vi "故障告警分析.vi"(8 "告警代码":u16, 9 "故障代码":u16, 10 "运行步序":u16, 11 "参数":string) -> (1 "告警记录":T1, 2 "故障记录":T1, 3 "简易报警状态":cluster{"故障状态":string, "报警状态":string})   [LabVIEW 2016, in "斯坦道总磷总氮V2.lvlib"]
panel:
  # "1、注射泵水样阀口堵塞；\n2、注射泵阀过载或丝杆无动作。"
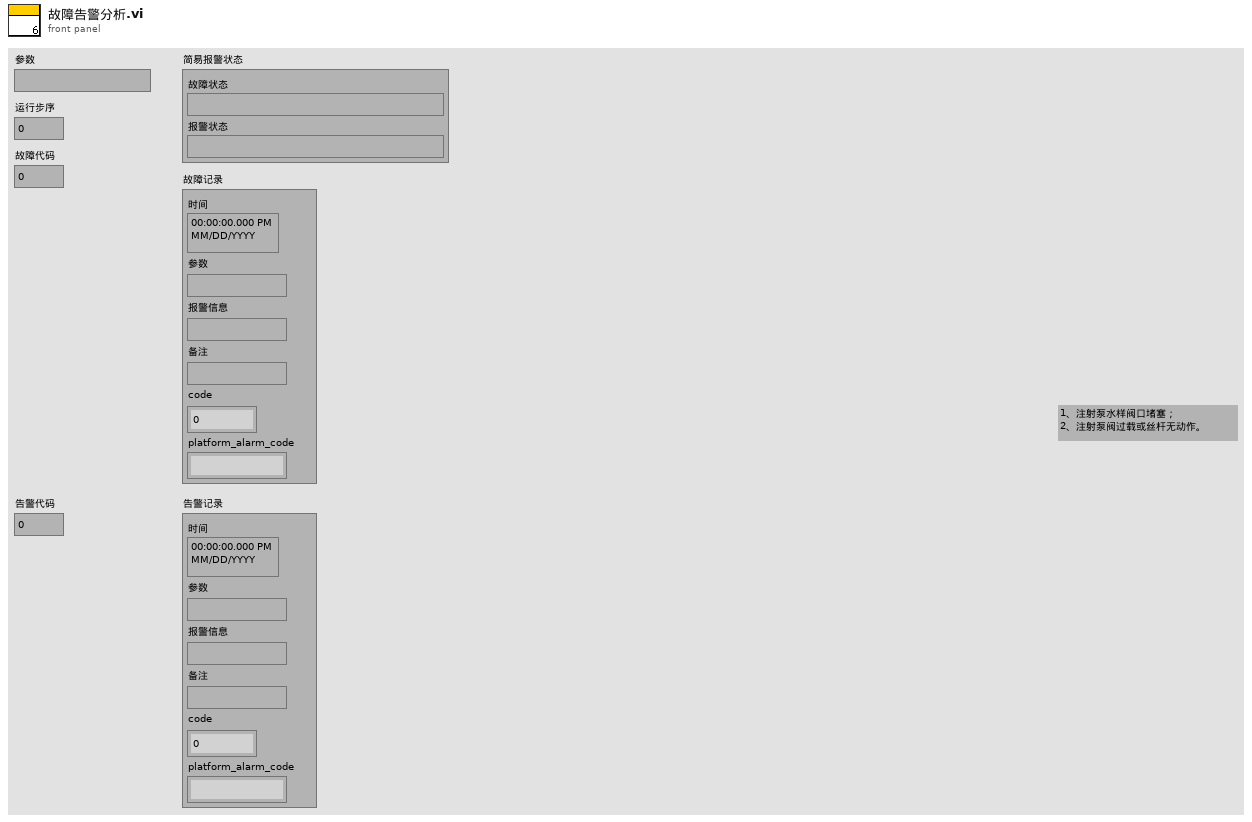
[diagram p1: front panel]
types:
  T1 = typedef "报警信息字段定义.ctl" = cluster{"时间":timestamp, "参数":string, "报警信息":string, "备注":string, "code":u64, "platform_alarm_code":string}
  T2 = cluster{"id":string, "ver":string, "type":string, "code":u16, "level":enum16{"一级", "二级", "三级"}, "message":string, "analysis":string, "platform_alarm_code":string}
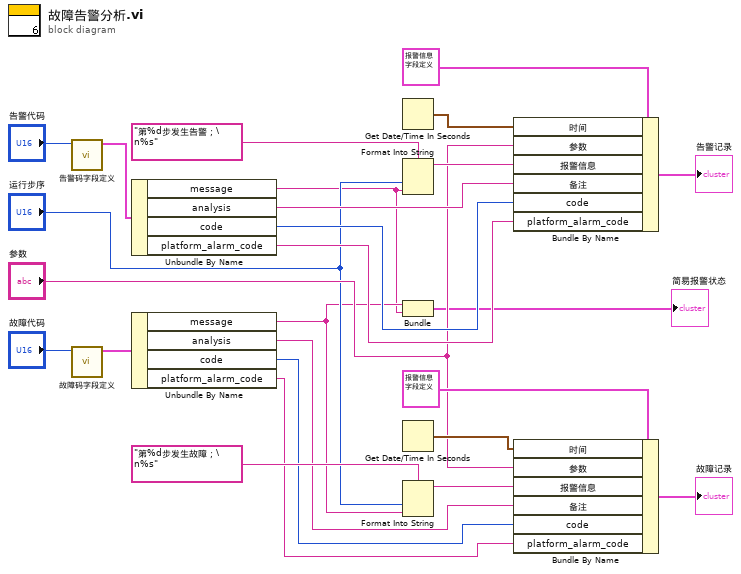
[diagram p0: block diagram]
diagram:
  n1 = call "告警码字段定义.vi"("告警代码"="告警代码") -> ("报警"=w6:T2)  [unwired: 10 in]
  n2 = call "故障码字段定义.vi"("故障代码"="故障代码") -> ("报警"=w23:T2)  [unwired: 10 in]
  n3 = Unbundle By Name(w6) -> ("message"=w2:string, "analysis"=w12:string, "code"=w13:u16, "platform_alarm_code"=w14:string)
  n4 = Unbundle By Name(w23) -> ("message"=w3:string, "analysis"=w17:string, "code"=w16:u16, "platform_alarm_code"=w15:string)
  n5 = Get Date/Time In Seconds() -> (seconds since 1Jan1904=w10:timestamp)
  n6 = Format Into String(format string="第%d步发生告警；\n%s" ("格式字符串"), "运行步序", w2) -> (resulting string=w11:string)  [unwired: 2 in, 1 out]
  n7 = Bundle("message"=w3, "message"=w2) -> (→"简易报警状态":cluster{"message":string, "message":string})  [unwired: 1 in]
  n8 = Get Date/Time In Seconds() -> (seconds since 1Jan1904=w19:timestamp)
  n9 = Format Into String(format string="第%d步发生故障；\n%s" ("格式字符串"), "运行步序", w3) -> (resulting string=w18:string)  [unwired: 2 in, 1 out]
  n10 = Bundle By Name(cluster=T1 {"时间"=timestamp(0 s since 1904-01-01), "参数"="", "报警信息"="", "备注"="", "code"=0, "platform_alarm_code"=""} ("故障记录"), "时间"=w10, "参数"="参数", "报警信息"=w11, "备注"=w12, "code"=w13, "platform_alarm_code"=w14) -> (→"告警记录":T1)
  n11 = Bundle By Name(cluster=T1 {"时间"=timestamp(0 s since 1904-01-01), "参数"="", "报警信息"="", "备注"="", "code"=0, "platform_alarm_code"=""} ("故障记录"), "时间"=w19, "参数"="参数", "报警信息"=w18, "备注"=w17, "code"=w16, "platform_alarm_code"=w15) -> (→"故障记录":T1)
